vi "MoveAxes.vi"(4 "Home":T3, 5 "Current Pulses In":dbl[](array[numeric]), 6 "Pos without backlash":bool, 7 "Current Pos In":dbl[](array[numeric]) format="%.2f", 8 "Channel Properties":T1[](array[typedef]) {"Current Pos" format="%.2f"; "Backlash/Eng units" format="%.2f"; "Pulses/rev" format="%.2f"; "Pos Tolerance" format="%.2f"; "Pulses/unit" format="%.2f"; "Acc. Min" format="%.2f"; "Acc. Max" format="%.2f"; "Vel. Min" format="%.2f"; "Vel. Max" format="%.2f"; "Acc. Default" format="%.2f"; "Vel. Default" format="%.2f"}, 9 "GoTo Array (Eng units all channels)":T4[](array[typedef]) {"Go To Position" step=100000.0}) -> (0 "Moved?":bool, 1 "Current Pos Out":dbl[](array[numeric]) format="%.2f", 2 "Error String":string, 3 "Current Pulses Out":dbl[](array[numeric]))   [LabVIEW 2022 SP3]
uses:
  ~subVIs/DriveGotoCluster.ctl
  Anemometry/Anemometry Sub Vis/Controls/Home.ctl
  ~subVIs/DriveProperties.ctl
  ~subVIs/Traverse Type.ctl
  ~subVIs/DriveClusterLower.ctl
  ~subVIs/GenericDriveCommand.ctl
  Anemometry/Anemometry Sub Vis/Globals/Trav_pos_global.vi
  ~subVIs/DriveConfigGlobal.vi
panel:
  out "Retry number":i32
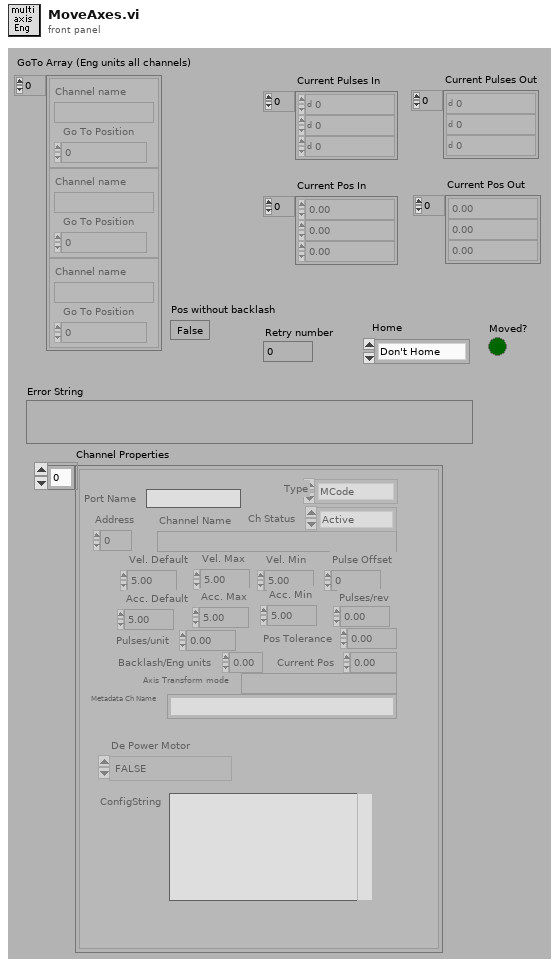
[diagram p1: front panel]
types:
  T1 = typedef "DriveProperties.ctl" = cluster{"Channel Name":string, "Vel. Default":sgl, "Acc. Default":sgl, "Vel. Max":sgl, "Vel. Min":sgl, "Acc. Max":sgl, "Acc. Min":sgl, "Pulses/unit":sgl, "Address":u8, "Pulse Offset":i32, "Pos Tolerance":sgl, "Pulses/rev":sgl, "Backlash/Eng units":sgl, "Current Pos":sgl, "Ch Status":enum16{"Active", "Offline", "Simulate"}, "Port Name":string, "Axis Transform mode":string, "Metadata Ch Name":string, "Type":T2, "De Power Motor":enum16{"TRUE", "FALSE"}, "ConfigString":string}
  T2 = typedef "Traverse Type.ctl" = enum16{"MCode", "Dynamixel"}
  T3 = typedef "Home.ctl" = enum16{"Don't Home", "Home  +X", "Home  -X", "Home  +Y", "Home  -Y", "Home  +Z", "Home  -Z"}
  T4 = typedef "DriveGotoCluster.ctl" = cluster{"Channel name":string, "Go To Position":dbl}
  T5 = typedef "GenericDriveCommand.ctl" = string
  T6 = cluster{"Total travel time":sgl, "Accel time":sgl, "Accel fractional distance":sgl}
  T7 = typedef "DriveClusterLower.ctl" = cluster{"Go To Position":dbl, "Velocity":dbl, "Acceleration":dbl, "Address":u8}
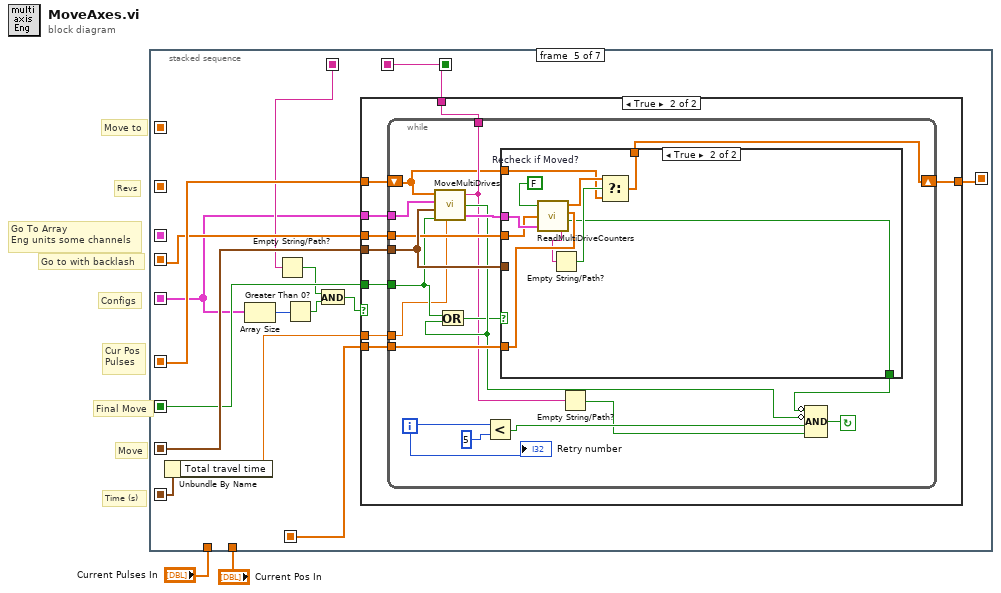
[diagram p0: block diagram]
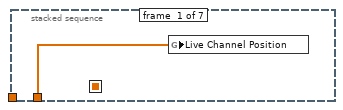
[diagram p2: hidden frame]
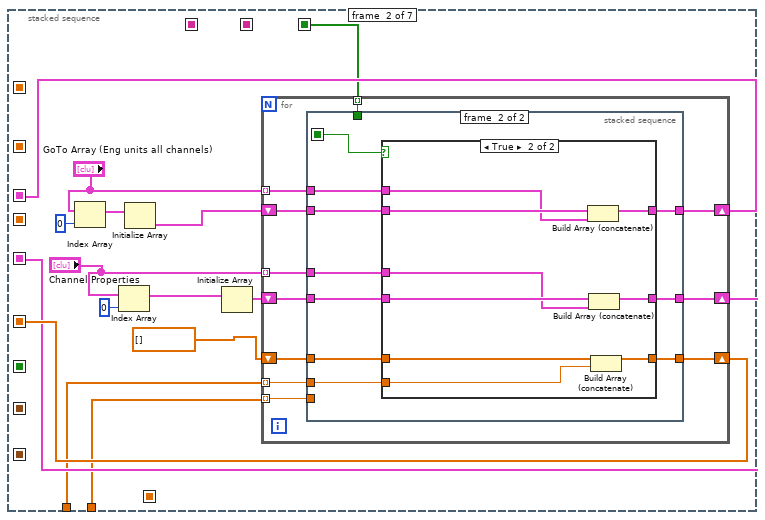
[diagram p3: hidden frame]
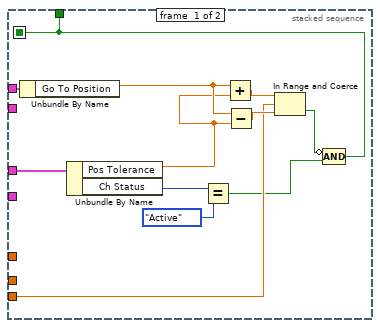
[diagram p4: hidden frame]
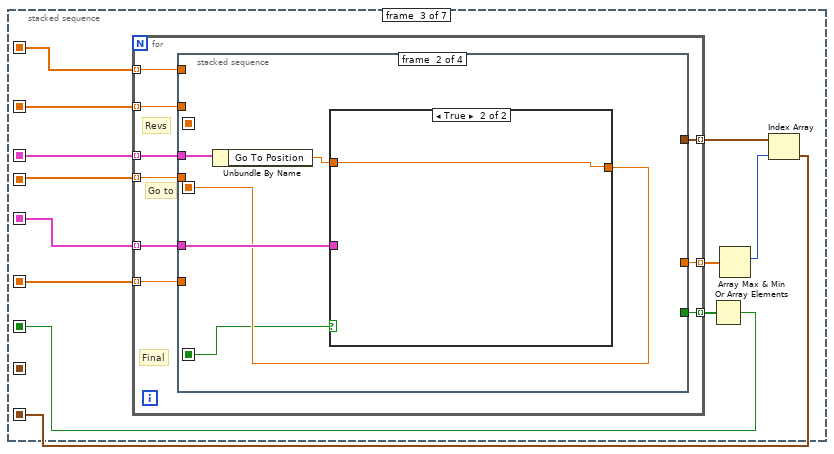
[diagram p6: hidden frame]
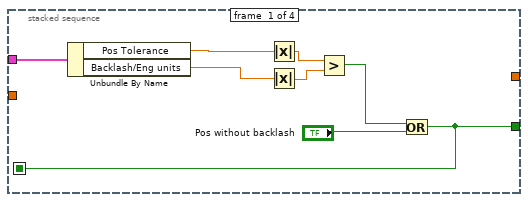
[diagram p7: hidden frame]
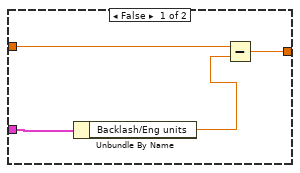
[diagram p8: hidden frame]
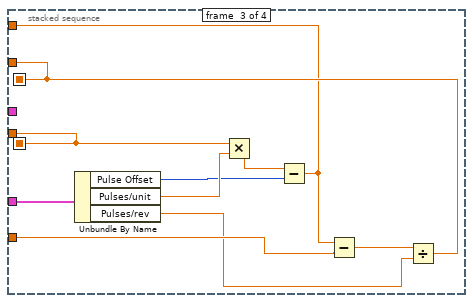
[diagram p9: hidden frame]
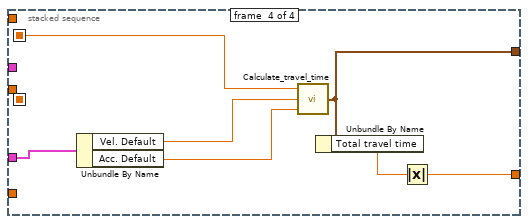
[diagram p10: hidden frame]
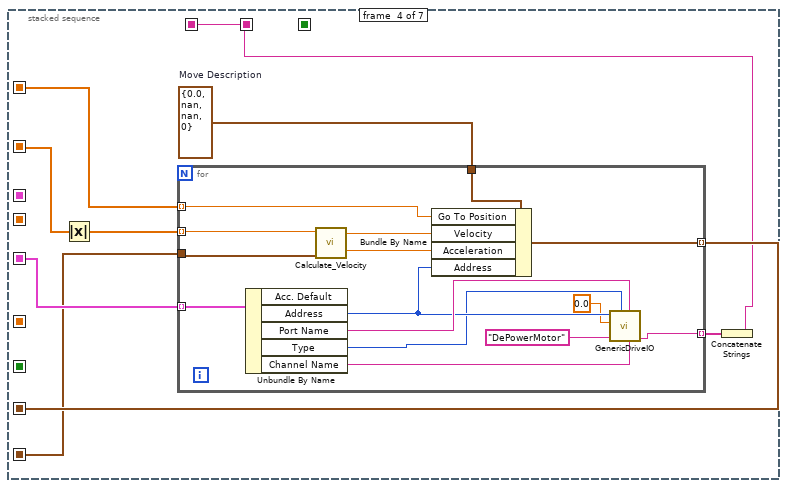
[diagram p11: hidden frame]
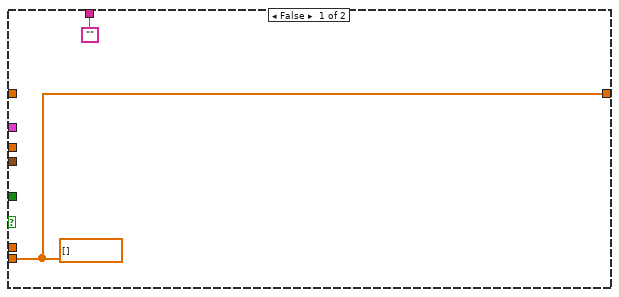
[diagram p12: hidden frame]
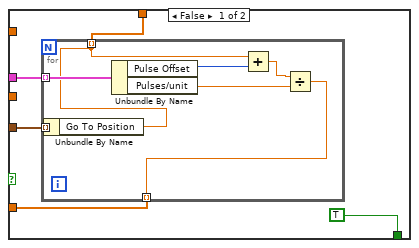
[diagram p13: hidden frame]
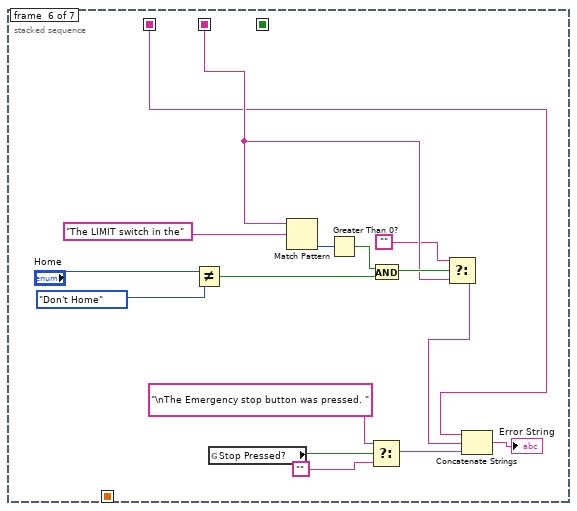
[diagram p14: hidden frame]
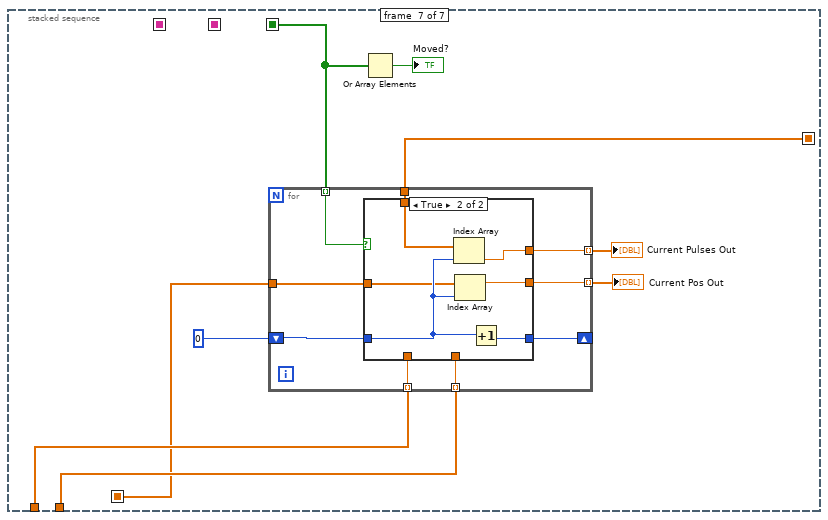
[diagram p15: hidden frame]
diagram:
  # "Go to with backlash"
  # "Final Move"
  # "Move"
  # "Cur Pos\nPulses"
  # "Configs"
  # "Go To Array\nEng units some channels"
  # "Revs"
  # "Move to"
  # "Time (s)"
  n1 = stacked-sequence {
    seq-local: [_ _ w64 _ _ _ _] -> [_ _ _ w122 w150 _ _]
    seq-local: [_ _ w74 _ _ _ _] -> [_ _ _ w127 _ _ _]
    seq-local: [_ _ w73 _ _ _ _] -> [_ _ _ w126 _ _ _]
    seq-local: [_ w9 _ _ _ _ _] -> [_ _ w71 _ _ _ _]
    seq-local: [_ w10 _ _ _ _ _] -> [_ _ w72 w125 w144 _ _]
    seq-local: [_ w11 _ _ _ _ _] -> [_ _ w70 _ w158 _ _]
    seq-local: [_ _ _ w124 _ _ _] -> [_ _ _ _ w157 _ _]
    seq-local: [_ _ _ _ w156 _ _] -> [_ _ _ _ _ _ w228]
    seq-local: [_ _ _ _ w155 _ _] -> [_ _ _ _ _ w216 _]
    seq-local: [_ w5 _ _ _ _ _] -> [_ _ _ _ _ _ w227]
    seq-local: [_ _ _ _ w154 _ _] -> [_ _ _ _ _ _ w229]
    seq-local: [_ _ w68 _ _ _ _] -> [_ _ _ _ w153 _ _]
    seq-local: [_ _ w67 _ _ _ _] -> [_ _ _ _ w152 _ _]
    seq-local: [_ _ _ w120 _ _ _] -> [_ _ _ _ w145 w210 _]
    tunnel: "Current Pulses In" -> [_ w7 _ _ _ _ w233]
    tunnel: "Current Pos In" -> [w3 w6 _ _ _ _ w231]
    frame #0 {
      n2 = global write "Trav_pos_global.vi" "Live Channel Position"(w3) -> ()
    }
    frame #1 {
      n3 = Index Array(array="GoTo Array (Eng units all channels)", index=0 ("Index")) -> (element=w16:T4)
      n4 = Index Array(array="Channel Properties", index=0 ("Index")) -> (element=w14:T1)
      n5 = Initialize Array(w16) -> (w15:T4[])  [unwired: 1 out]
      n6 = Initialize Array(w14) -> (w12:T1[])  [unwired: 1 out]
      n7 = for {
        tunnel: "Channel Properties" -> [w29] mode=indexing
        tunnel: "GoTo Array (Eng units all channels)" -> [w28] mode=indexing
        tunnel: w6 -> [w27] mode=indexing
        shift-right: [w23] -> w9
        shift-left: w15 -> [w24]
        shift-right: [w25] -> w10
        shift-left: w12 -> [w26]
        shift-right: [w21] -> w11
        shift-left: dbl[] [] -> [w22]
        tunnel: w7 -> [w20] mode=indexing
        tunnel: [w19] -> w5 mode=indexing
        n8 = stacked-sequence {
          seq-local: [w34 _] -> [_ w51]
          tunnel: w29 -> [w40 w48]
          tunnel: w28 -> [w41 w45]
          tunnel: w27 -> [w36 _]
          tunnel: w26 -> [_ w50]
          tunnel: [_ w49] -> w25
          tunnel: w24 -> [_ w47]
          tunnel: [_ w46] -> w23
          tunnel: w22 -> [_ w44]
          tunnel: [_ w43] -> w21
          tunnel: w20 -> [_ w42]
          tunnel: [w34 _] -> w19
          frame #0 {
            n9 = Unbundle By Name(w41) -> ("Go To Position"=w39:dbl)
            n10 = Unbundle By Name(w40) -> ("Pos Tolerance"=w33:sgl, "Ch Status"=w32:enum16{"Active", "Offline", "Simulate"})
            n11 = Equal?(x=w32, y=enum16{"Active", "Offline", "Simulate"}."Active" ("Channel Properties.Ch Status")) -> (x = y?=w30:bool)
            n12 = Add(x=w39, y=w33) -> (x+y=w38:dbl)
            n13 = Subtract(x=w39, y=w33) -> (x-y=w37:dbl)
            n14 = In Range and Coerce(upper limit=w38, x=w36, lower limit=w37) -> (In Range?=w35:bool)  [unwired: 1 out]
            n15 = Compound Arithmetic op=AND(invert w35, w30) -> (w34:bool)
          }
          frame #1 {
            n16 = case shown="True" w51 {
              tunnel: w50 -> [w53 w63]
              tunnel: [w53 w62] -> w49
              tunnel: w48 -> [_ w61]
              tunnel: w47 -> [w54 w60]
              tunnel: [w54 w59] -> w46
              tunnel: w45 -> [_ w58]
              tunnel: w44 -> [w52 w57]
              tunnel: [w52 w56] -> w43
              tunnel: w42 -> [_ w55]
              frame False {
              }
              frame True {
                n17 = Build Array (concatenate)(w60, w58) -> (w59:T4[])
                n18 = Build Array (concatenate)(w63, w61) -> (w62:T1[])
                n19 = Build Array (concatenate)(w57, w55) -> (w56:dbl[])
              }
            }
          }
        }
      }
    }
    frame #2 {
      n20 = for {
        tunnel: w72 -> [w84] mode=indexing
        tunnel: w71 -> [w83] mode=indexing
        tunnel: w70 -> [w82] mode=indexing
        tunnel: [w81] -> w75 mode=indexing
        tunnel: [w80] -> w74 mode=indexing
        tunnel: [w79] -> w73 mode=indexing
        tunnel: [w78] -> w69 mode=indexing
        tunnel: [w77] -> w67 mode=indexing
        tunnel: [w76] -> w66 mode=indexing
        # "Final"
        # "Go to"
        # "Revs"
        n21 = stacked-sequence {
          seq-local: [_ _ w109 _] -> [_ _ _ w115]
          seq-local: [_ w94 _ _] -> [_ _ w103 _]
          seq-local: [w85 _ _ _] -> [_ w93 _ _]
          tunnel: w84 -> [w92 w96 w111 w119]
          tunnel: w83 -> [_ w97 _ _]
          tunnel: w82 -> [_ _ w110 _]
          tunnel: [_ _ _ w118] -> w81
          tunnel: [_ _ w106 _] -> w80
          tunnel: [_ _ w109 _] -> w79
          tunnel: [w85 _ _ _] -> w78
          tunnel: [_ _ w103 _] -> w77
          tunnel: [_ _ _ w114] -> w76
          frame #0 {
            n22 = Unbundle By Name(w92) -> ("Pos Tolerance"=w91:sgl, "Backlash/Eng units"=w90:sgl)
            n23 = Absolute Value(x=w91) -> (abs(x)=w89:sgl)
            n24 = Absolute Value(x=w90) -> (abs(x)=w88:sgl)
            n25 = Greater?(x=w89, y=w88) -> (0:w87:bool)
            n26 = Or(x=w87, y="Pos without backlash") -> (x .or. y?=w85:bool)
          }
          frame #1 {
            n27 = Unbundle By Name(w97) -> ("Go To Position"=w95:dbl)
            n28 = case shown="True" w93 {
              tunnel: w96 -> [w101 _]
              tunnel: w95 -> [w99 w102]
              tunnel: [w98 w102] -> w94
              frame False {
                n29 = Unbundle By Name(w101) -> ("Backlash/Eng units"=w100:sgl)
                n30 = Subtract(x=w99, y=w100) -> (x-y=w98:dbl)
              }
              frame True {
              }
            }
          }
          frame #2 {
            n31 = Unbundle By Name(w111) -> ("Pulse Offset"=w104:i32, "Pulses/unit"=w112:sgl, "Pulses/rev"=w107:sgl)
            n32 = Multiply(x=w103, y=w112) -> (x*y=w105:dbl)
            n33 = Subtract(x=w105, y=w104) -> (x-y=w106:dbl)
            n34 = Subtract(x=w106, y=w110) -> (x-y=w108:dbl)
            n35 = Divide(x=w108, y=w107) -> (x/y=w109:dbl)
          }
          frame #3 {
            n36 = Unbundle By Name(w119) -> ("Vel. Default"=w116:sgl, "Acc. Default"=w117:sgl)
            n37 = call "Calculate_travel_time.vi"("Default Acceleration Revs/s^2"=w117, "Default Velocity Revs/s"=w116, "Revs to travel"=w115) -> ("Times"=w114:T6)
            n38 = Unbundle By Name(w114) -> ("Total travel time"=w113:sgl)
            n39 = Absolute Value(x=w113) -> (abs(x)=w118:sgl)
          }
        }
      }
      n40 = Or Array Elements(Boolean array=w69) -> (logical OR=w68:bool)
      n41 = Array Max & Min(array=w75) -> (max index (indices)=w65:i32)  [unwired: 3 out]
      n42 = Index Array(array=w66, index=w65) -> (element=w64:T6)
    }
    frame #3 {
      w128 = T7 {"Go To Position"=0.0, "Velocity"=nan, "Acceleration"=nan, "Address"=0}  # Move Description
      n43 = Absolute Value(x=w126) -> (abs(x)=w123:dbl[])
      n44 = for {
        tunnel: w128 -> [w143]
        tunnel: w127 -> [w138] mode=indexing
        tunnel: w125 -> [w142] mode=indexing
        tunnel: w123 -> [w139] mode=indexing
        tunnel: [w141] -> w124 mode=indexing
        tunnel: w122 -> [w134]
        tunnel: [w129] -> w121 mode=indexing
        n45 = Unbundle By Name(w142) -> ("Address"=w136:u8, "Port Name"=w140:string, "Type"=w132:T2, "Channel Name"=w133:string)  [unwired: 1 out]
        n46 = call "Calculate_Velocity.vi"("Times"=w134, "Revs to travel"=w139) -> ("Acceleration"=w135:dbl, "Max Velocity"=w137:dbl)  [unwired: 1 in, 1 out]
        n47 = Bundle By Name(cluster=w143, "Go To Position"=w138, "Velocity"=w137, "Acceleration"=w135, "Address"=w136) -> (w141:T7)
        n48 = call "GenericDriveIO.vi"("GenericDriveCommand"=T5 "DePowerMotor", "Channel Name"=w133, "Numeric Value"=0.0, "Address"=w136, "Type"=w132, "Port Name"=w140) -> ("Error Description"=w129:string)  [unwired: 1 in, 4 out]
      }
      n49 = Concatenate Strings(w121) -> (w120:string)
    }
    frame #4 {
      n50 = Unbundle By Name(w150) -> ("Total travel time"=w149:sgl)
      n51 = Array Size(array=w144) -> (size(s)=w151:i32)
      n52 = Empty String/Path?(string/path=w145) -> (empty?=w146:bool)
      n53 = Greater Than 0?(x=w151) -> (x > 0?=w148:bool)
      n54 = And(x=w146, y=w148) -> (x .and. y?=w147:bool)
      n55 = case shown="True" w147 {
        tunnel: w158 -> [_ w169]
        tunnel: w144 -> [_ w168]
        tunnel: w157 -> [_ w167]
        tunnel: [w159 w166] -> w156
        tunnel: ["" w165] -> w155
        tunnel: [w159 w164] -> w154
        tunnel: w153 -> [_ w163]
        tunnel: w152 -> [_ w162]
        tunnel: w149 -> [_ w161]
        frame False {
          w159 = dbl[] [] ("Eng units")
        }
        frame True {
          n56 = while {
            tunnel: w161 -> [w171]
            tunnel: w162 -> [w178]
            tunnel: [w174] -> w165
            tunnel: w163 -> [w172]
            tunnel: [w183] -> w166
            shift-left: w169 -> [w170]
            shift-right: [w182] -> w164
            tunnel: w168 -> [w181]
            tunnel: w167 -> [w179]
            i -> [w187]
            stop <- w184 continue-if-true
            n57 = call "MoveMultiDrives.vi"("Start Counter"=w170, "Channel Properties"=w181, "GoTo Array (pulse position, some channels)"=w179, "Final move"=w172, "Predicted Move Time"=w171) -> ("Error string"=w174:string, "Stop Pressed?"=w177:bool, "Channel Properties Out"=w180:T1[])
            n58 = Or(x=w172, y=w177) -> (x .or. y?=w176:bool)
            n59 = Less?(x=w187, y=5) -> (x < y?=w185:bool)
            n60 = case shown="True" w176 {
              tunnel: w179 -> [w191 _]
              tunnel: [TRUE w200] -> w175
              tunnel: [w190 w209] -> w183
              tunnel: [w188 w202] -> w182
              tunnel: w180 -> [w189 w208]
              tunnel: w178 -> [_ w201]
              tunnel: w170 -> [_ w203]
              frame False {
                n61 = for {
                  tunnel: w191 -> [w199] mode=indexing
                  tunnel: [w196] -> w190 mode=indexing
                  tunnel: w189 -> [w198] mode=indexing
                  tunnel: [w194] -> w188 mode=indexing
                  n62 = Unbundle By Name(w199) -> ("Go To Position"=w194:dbl)
                  n63 = Unbundle By Name(w198) -> ("Pulse Offset"=w195:i32, "Pulses/unit"=w197:sgl)
                  n64 = Add(x=w194, y=w195) -> (x+y=w193:dbl)
                  n65 = Divide(x=w193, y=w197) -> (x/y=w196:dbl)
                }
              }
              frame True {
                w207 = FALSE  # Recheck if Moved?
                n66 = call "ReadMultiDriveCounters.vi"("Recheck if Moved?"=w207, "Position input XYZ"=w201, "Channel Properties"=w208) -> ("Pulses"=w204:sgl[], "Eng units"=w209:sgl[], "Position Correct"=w200:bool, "Error String"=w206:string)
                n67 = Empty String/Path?(string/path=w206) -> (empty?=w205:bool)
                n68 = Select(t=w204, s=w205, f=w203) -> (s? t:f=w202:dbl[])
              }
            }
            n69 = Empty String/Path?(string/path=w174) -> (empty?=w173:bool)
            n70 = Compound Arithmetic op=AND(invert w175, invert w177, w185, w173) -> (w184:bool)
            "Retry number" <- w187
          }
        }
      }
    }
    frame #5 {
      n71 = Not Equal?(x="Home", y=Home."Don't Home" ("Home")) -> (x != y?=w211:bool)
      n72 = global read "DriveConfigGlobal.vi" "Stop Pressed?"() -> (w225:bool)
      n73 = Match Pattern(string=w216, regular expression="The LIMIT switch in the") -> (offset past match=w219:i32)  [unwired: 1 in, 3 out]
      n74 = Greater Than 0?(x=w219) -> (x > 0?=w218:bool)
      n75 = Select(t="\nThe Emergency stop button was pressed. ", s=w225, f="") -> (s? t:f=w222:string)
      n76 = And(x=w218, y=w211) -> (x .and. y?=w217:bool)
      n77 = Select(t="", s=w217, f=w216) -> (s? t:f=w215:string)
      n78 = Concatenate Strings(w210, w215, w222) -> (→"Error String":string)
    }
    frame #6 {
      n79 = for {
        shift-right: [w238] -> _
        shift-left: 0 -> [w237]
        tunnel: w227 -> [w243] mode=indexing
        tunnel: w233 -> [w242] mode=indexing
        tunnel: [w241] -> w232 mode=indexing
        tunnel: w231 -> [w240] mode=indexing
        tunnel: [w239] -> w230 mode=indexing
        tunnel: w229 -> [w236]
        tunnel: w228 -> [w235]
        n80 = case shown="True" w243 {
          tunnel: w242 -> [w246 _]
          tunnel: [w246 w250] -> w241
          tunnel: w240 -> [w245 _]
          tunnel: [w245 w249] -> w239
          tunnel: [w244 w252] -> w238
          tunnel: w237 -> [w244 w251]
          tunnel: w236 -> [_ w248]
          tunnel: w235 -> [_ w247]
          frame False {
          }
          frame True {
            n81 = Index Array(array=w248, index=w251) -> (element=w250:dbl)
            n82 = Index Array(array=w247, index=w251) -> (element=w249:dbl)
            n83 = Increment(x=w251) -> (x+1=w252:i32)
          }
        }
      }
      "Current Pulses Out" <- w232
      "Current Pos Out" <- w230
      n84 = Or Array Elements(Boolean array=w227) -> (logical OR=→"Moved?":bool)
    }
  }
